vi "assembly_I_SET_command.vi"(8 "error_in":errorcluster, 10 "curr":dbl=0.001 min=0.001 max=0.999, 11 "channel":T1=enum."1") -> (0 "error_out":errorcluster, 3 "command":string)   [LabVIEW 2017]
uses:
  types/channels_enum.ctl
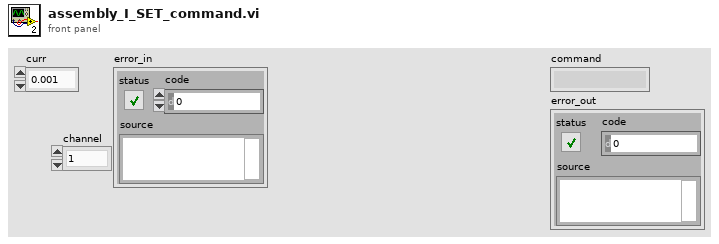
[diagram p1: front panel]
types:
  T1 = typedef "channels_enum.ctl" = enum16{"0", "1", "2"}
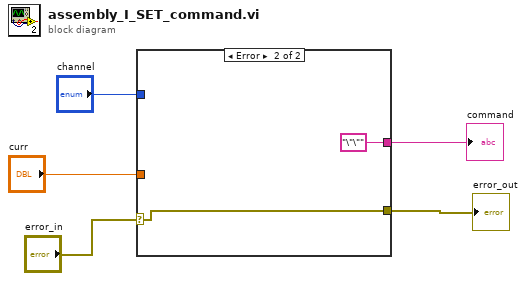
[diagram p0: block diagram]
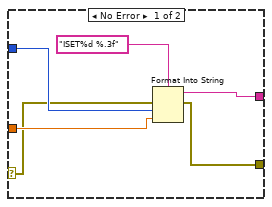
[diagram p2: hidden frame]
diagram:
  n1 = case shown="Error" "error_in" {
    selector: "error_in" -> [w7 w12]
    tunnel: "curr" -> [w11 _]
    tunnel: [w9 "\"\""] -> w4
    tunnel: "channel" -> [w8 _]
    tunnel: [w6 w12] -> w2
    frame No Error {
      n2 = Format Into String(format string="ISET%d %.3f", error in=w7, w8, w11) -> (resulting string=w9:string, error out=w6:errorcluster)  [unwired: 1 in]
    }
    frame Error {
    }
  }
  "command" <- w4
  "error_out" <- w2
